vi "HK Channel Get Current Values.vi"(8 "error in (no error)":errorcluster, 11 "HK Channel in":refnum<class "HK Table.lvclass">) -> (0 "error out":errorcluster, 1 "Times and values":cluster{"Time Stamp":timestamp, "Value":dbl}[](array[cluster]), 2 "Names":string[](array[string]), 3 "HK Channel out":refnum<class "HK Table.lvclass">)   [LabVIEW 2019, in "HK Table.lvclass"]
uses:
  HK Table.lvclass
  HK Table.lvclass/HK Table.ctl
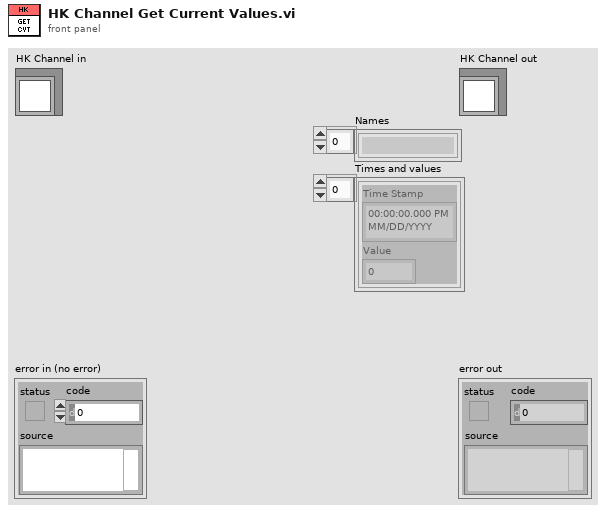
[diagram p1: front panel]
types:
  T1 = typedef "HK Table.lvclass/HK Current Value Table Element.ctl" = cluster{"Value":dbl, "Time Stamp":timestamp, "Running Avg.":dbl, "Std. Dev.":dbl, "Recent Values":dbl[], "Timestamps":timestamp[], "Alarm Status":T2}
  T2 = typedef "HK Item.lvclass/HK Alarm enum Status.ctl" = enum16{"No Alarm", "Red Low", "Red High", "Yellow Low", "Yellow High"}
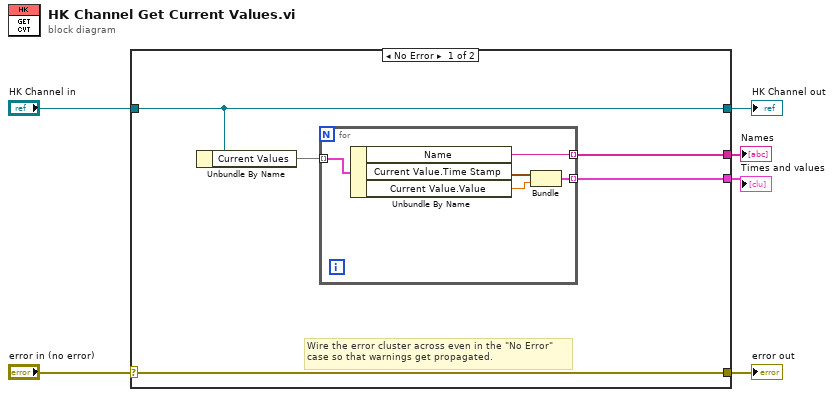
[diagram p0: block diagram]
diagram:
  n1 = case shown="No Error" "error in (no error)" {
    selector: "error in (no error)" -> [w11 w18]
    tunnel: [w11 w18] -> w5
    tunnel: [w10 w17] -> w3
    tunnel: "HK Channel in" -> [w10 w17]
    tunnel: [w8 _] -> w2
    tunnel: [w7 _] -> w1
    frame No Error {
      # "Wire the error cluster across even in the \"No Error\"\ncase so that warnings get propagated."
      n2 = Unbundle By Name(w10) -> ("Current Values"=w9:map{string, T1})
      n3 = for {
        tunnel: w9 -> [w16] mode=indexing
        tunnel: [w15] -> w8 mode=indexing
        tunnel: [w12] -> w7 mode=indexing
        n4 = Unbundle By Name(w16) -> ("Name"=w15:string, "Current Value.Time Stamp"=w14:timestamp, "Current Value.Value"=w13:dbl)
        n5 = Bundle("Time Stamp"=w14, "Value"=w13) -> (w12:cluster{"Time Stamp":timestamp, "Value":dbl})  [unwired: 1 in]
      }
    }
    frame Error {
    }
  }
  "error out" <- w5
  "HK Channel out" <- w3
  "Names" <- w2
  "Times and values" <- w1
